vi "solar_addon QTimers.vi"(11 "Variant":variant) -> (0 "error out":errorcluster)   [LabVIEW 2018]
doc: "This SOLAR addon configures the QTimer periodic messaging interface."
uses:
  solar/solar_ctl SOLAR Refnum.ctl
panel:
  in  "Export":bool
  in  "Apply":bool
  in  "Stop All":bool
  out "Destination Queue":string
  in  "Add":bool
  in  "Messages":string
  out "Messages to Enqueue":cluster{"MSG":string, "DATA":variant}[](array[cluster])
  in  "Stop":bool
  in  "Start":bool
  in  "EnQ_Type":enum8{"Normal", "Priority", "IgnoreIfExists"}(ring)
  out "Running":bool
  in  "Delay":i32 format="%d ms"
  out "QTimer":string
  in  "QTimersLB":i32(listbox)
  in  "Refresh":bool
  # "CMD{TYPE:VALUE,...}"
  # "Ex: READ{i32:123,bool:true,str:'test'}"
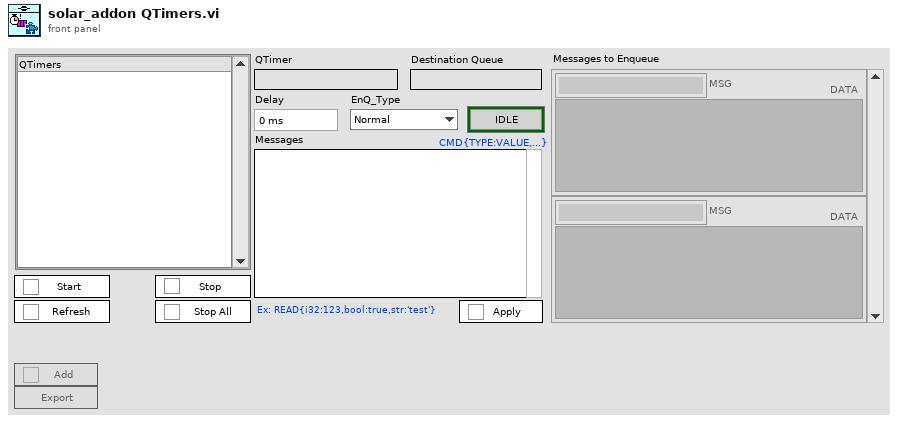
[diagram p1: front panel]
types:
  T1 = typedef "solar_ctl SOLAR Refnum.ctl" = refnum<k1>
  T2 = cluster{"image type":i32, "image depth":i32, "image":u8[], "mask":u8[], "colors":u32[], "Rectangle":cluster{"left":i16, "top":i16, "right":i16, "bottom":i16}}[]
  T3 = typedef "solar_ctl SOLAR Global.ctl" = cluster{"Targets":T4[], "AppDir":path, "solar.ini":path, "ConfigsDir":path, "CosmosDir":path, "LogsDir":path, "ExePath":path, "ExeVersion":string, "PartNum":string, "AppSetup":string, "Title":string, "Main.ini":path, "Temp.ini":path, "vSOLAR":string, "Splash.png":string, "SplashWait":i32, "SOLARUE":refnum<user-event>, "VoyagerRefnum":T5, "QTimerRefnum":T6}
  T4 = typedef "solar_ctl Target Global.ctl" = cluster{"Target":string, "Q":refnum<queue>, "UE":refnum<user-event>, "VI":refnum<vi>, "Menu":refnum<k9>, "Data":refnum<data-value>, "Attributes":variant}
  T5 = typedef "solar_voy_ctl Voyager Refnum.ctl" = refnum<k1>
  T6 = typedef "solar_qtimer_ctl Refnum.ctl" = refnum<k1>
  T7 = typedef "solar_qtimer_ctl QTimer.ctl" = cluster{"Settings":T8, "Queue":refnum<queue>, "QTimerQ":refnum<queue>, "VI Refnum":refnum<vi>}
  T8 = typedef "solar_qtimer_ctl QTimer Settings.ctl" = cluster{"QTimer":string, "Delay":i32, "Start":bool, "EnQ_Type":enum8{"Normal", "Priority", "IgnoreIfExists"}, "Messages":cluster{"MSG":string, "DATA":variant}[]}
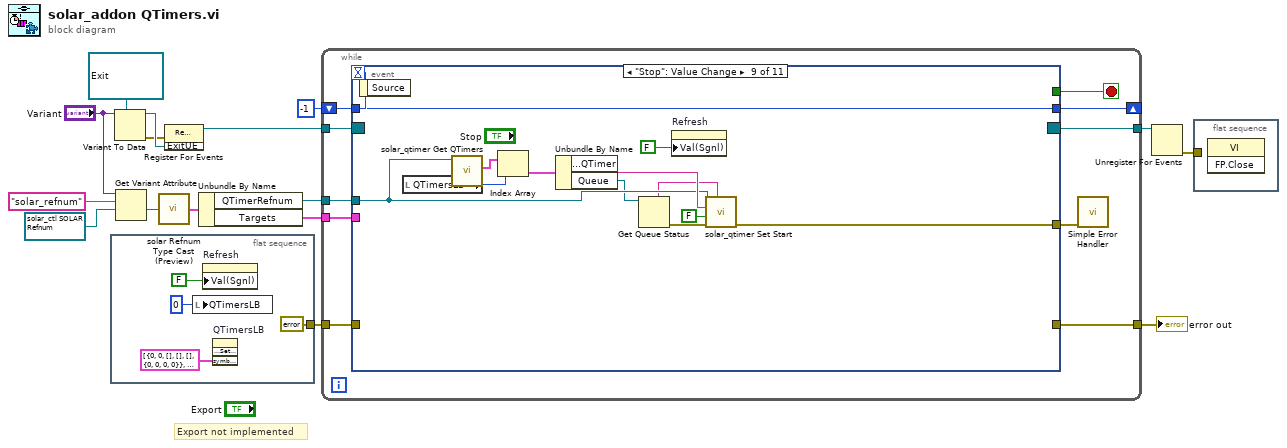
[diagram p0: block diagram]
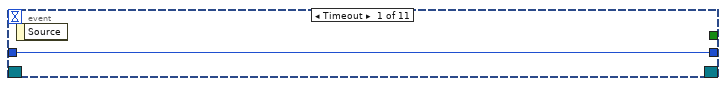
[diagram p2: hidden frame]
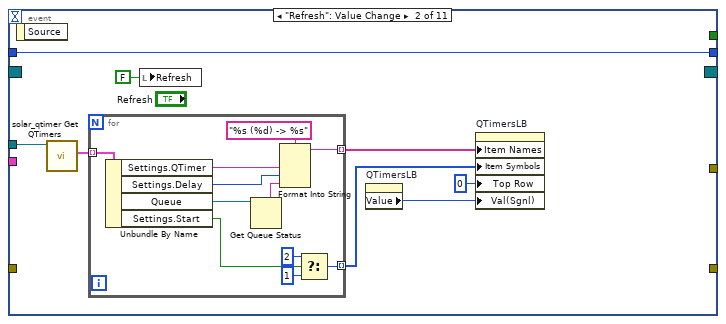
[diagram p3: hidden frame]
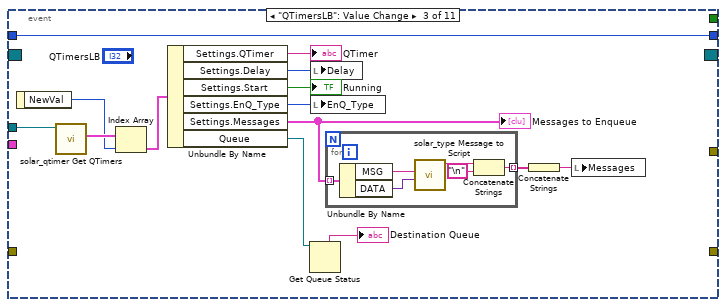
[diagram p4: hidden frame]
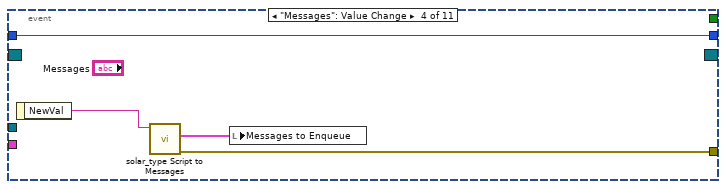
[diagram p5: hidden frame]
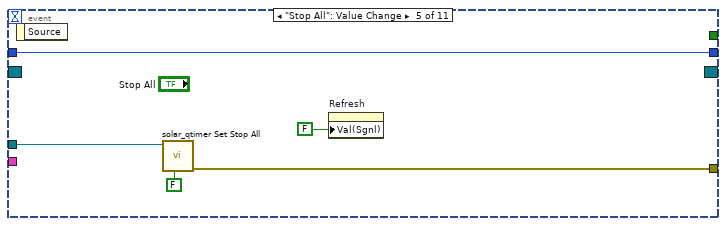
[diagram p6: hidden frame]
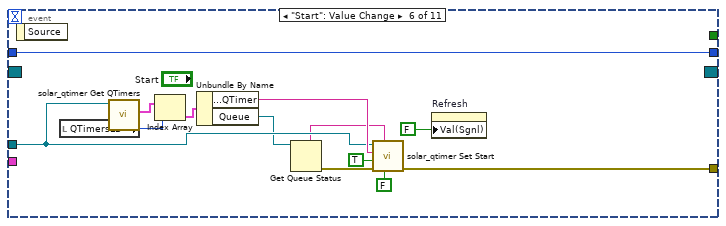
[diagram p7: hidden frame]
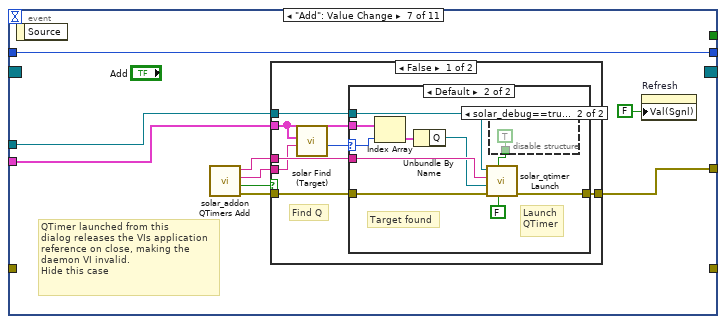
[diagram p8: hidden frame]
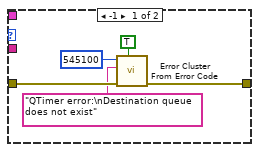
[diagram p9: hidden frame]
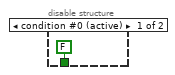
[diagram p10: hidden frame]
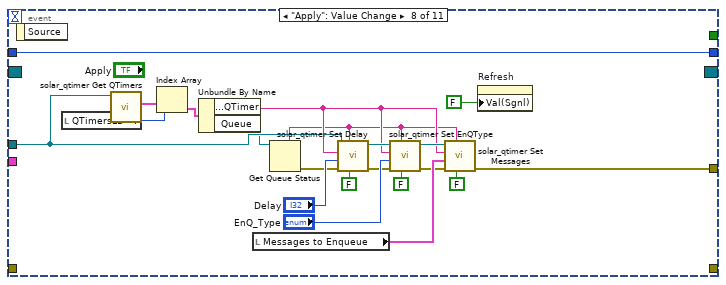
[diagram p12: hidden frame]
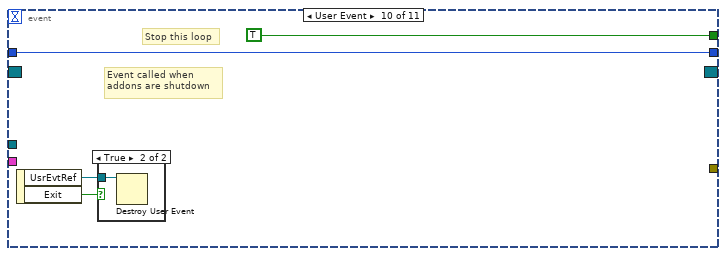
[diagram p13: hidden frame]
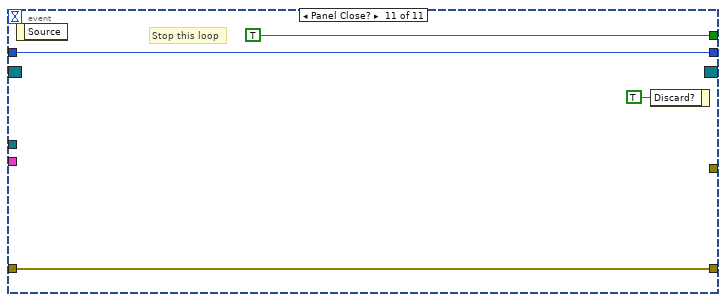
[diagram p15: hidden frame]
diagram:
  w11 = T1 refnum items=["solar"] ("SOLAR Refnum")
  # "Export not implemented"
  n1 = flat-sequence {
    tunnel: [errorcluster {"status"=FALSE, "code"=0, "source"=""} ("error in (no error)")] -> w1
    frame #0 {
      n2 = local write "QTimersLB"(0 ("QTimersLB")) -> ()
      n3 = property on="Refresh" class="Bool (strict)"("Val(Sgnl)"=FALSE ("Update")) -> ()  [unwired: 2 in, 2 out]
      n4 = invoke on="QTimersLB" class="LstBox (strict)" method="Custom Item Symbols.Set Symbol Array"("symbols"=T2 [{"image type"=0, "image depth"=0, "image"=[], "mask"=[], "colors"=[], "Rectangle"={"left"=0, "top"=0, "right"=0, "bottom"=0}}, {"image type"=0, "image depth"=32, "image"=[0, 0, 0, 0, 0, 0, 0, 0, 0, 0, 0, 0, 0, 0, 0, 0, 0, 0, 0, 0, 0, 0, 0, 0, 0, 0, 0, 0, 0, 0, 0, 0, 0, 0, 0, 0, 0, 0, 0, 0, 0, 0, 0, 0, 0, 0, 0, 0, 0, 0, 0, 0, 0, 0, 0, 0, 0, 0, 0, 0, 0, 0, 0, 0, 0, 0, 0, 0, 0, 0, 0, 0, 0, 0, 0, 0, 0, 0, 0, 0, 0, 0, 0, 0, 0, 0, 0, 0, 0, 0, 0, 0, 0, 0, 0, 0, 0, 0, 0, 0, 0, 0, 0, 0, 0, 0, 0, 0, 0, 0, 0, 0, 0, 0, 0, 0, 0, 0, 0, 0, 0, 0, 0, 0, 0, 0, 0, 0, 0, 0, 0, 0, 0, 0, 0, 0, 255, 157, 0, 0, 255, 157, 0, 0, 255, 157, 0, 0, 255, 157, 0, 0, 255, 157, 0, 0, 255, 157, 0, 0, 255, 157, 0, 0, 255, 157, 0, 0, 255, 157, 0, 0, 255, 157, 0, 0, 255, 157, 0, 0, 255, 157, 0, 0, 0, 0, 0, 0, 0, 0, 0, 0, 0, 0, 0, 0, 0, 0, 0, 0, 255, 157, 0, 0, 255, 247, 0, 0, 255, 247, 0, 0, 255, 247, 0, 0, 255, 247, 0, 0, 255, 247, 0, 0, 255, 247, 0, 0, 255, 247, 0, 0, 255, 247, 0, 0, 255, 247, 0, 0, 255, 247, 0, 0, 255, 157, 0, 0, 0, 0, 0, 0, 0, 0, 0, 0, 0, 0, 0, 0, 0, 0, 0, 0, 255, 157, 0, 0, 255, 240, 0, 0, 255, 240, 0, 0, 255, 240, 0, 0, 255, 240, 0, 0, 255, 240, 0, 0, 255, 240, 0, 0, 255, 240, 0, 0, 255, 240, 0, 0, 255, 240, 0, 0, 255, 240, 0, 0, 255, 157, 0, 0, 0, 0, 0, 0, 0, 0, 0, 0, 0, 0, 0, 0, 0, 0, 0, 0, 255, 157, 0, 0, 255, 232, 0, 0, 255, 232, 0, 0, 255, 232, 0, 0, 255, 232, 0, 0, 255, 232, 0, 0, 255, 232, 0, 0, 255, 232, 0, 0, 255, 232, 0, 0, 255, 232, 0, 0, 255, 232, 0, 0, 255, 157, 0, 0, 0, 0, 0, 0, 0, 0, 0, 0, 0, 0, 0, 0, 0, 0, 0, 0, 255, 157, 0, 0, 255, 225, 0, 0, 255, 225, 0, 0, 255, 225, 0, 0, 255, 225, 0, 0, 255, 225, 0, 0, 255, 225, 0, 0, 255, 225, 0, 0, 255, 225, 0, 0, 255, 225, 0, 0, 255, 225, 0, 0, 255, 157, 0, 0, 0, 0, 0, 0, 0, 0, 0, 0, 0, 0, 0, 0, 0, 0, 0, 0, 255, 157, 0, 0, 255, 217, 0, 0, 255, 217, 0, 0, 255, 217, 0, 0, 255, 217, 0, 0, 255, 217, 0, 0, 255, 217, 0, 0, 255, 217, 0, 0, 255, 217, 0, 0, 255, 217, 0, 0, 255, 217, 0, 0, 255, 157, 0, 0, 0, 0, 0, 0, 0, 0, 0, 0, 0, 0, 0, 0, 0, 0, 0, 0, 255, 157, 0, 0, 255, 210, 0, 0, 255, 210, 0, 0, 255, 210, 0, 0, 255, 210, 0, 0, 255, 210, 0, 0, 255, 210, 0, 0, 255, 210, 0, 0, 255, 210, 0, 0, 255, 210, 0, 0, 255, 210, 0, 0, 255, 157, 0, 0, 0, 0, 0, 0, 0, 0, 0, 0, 0, 0, 0, 0, 0, 0, 0, 0, 255, 157, 0, 0, 255, 202, 0, 0, 255, 202, 0, 0, 255, 202, 0, 0, 255, 202, 0, 0, 255, 202, 0, 0, 255, 202, 0, 0, 255, 202, 0, 0, 255, 202, 0, 0, 255, 202, 0, 0, 255, 202, 0, 0, 255, 157, 0, 0, 0, 0, 0, 0, 0, 0, 0, 0, 0, 0, 0, 0, 0, 0, 0, 0, 255, 157, 0, 0, 255, 195, 0, 0, 255, 195, 0, 0, 255, 195, 0, 0, 255, 195, 0, 0, 255, 195, 0, 0, 255, 195, 0, 0, 255, 195, 0, 0, 255, 195, 0, 0, 255, 195, 0, 0, 255, 195, 0, 0, 255, 157, 0, 0, 0, 0, 0, 0, 0, 0, 0, 0, 0, 0, 0, 0, 0, 0, 0, 0, 255, 157, 0, 0, 255, 187, 0, 0, 255, 187, 0, 0, 255, 187, 0, 0, 255, 187, 0, 0, 255, 187, 0, 0, 255, 187, 0, 0, 255, 187, 0, 0, 255, 187, 0, 0, 255, 187, 0, 0, 255, 187, 0, 0, 255, 157, 0, 0, 0, 0, 0, 0, 0, 0, 0, 0, 0, 0, 0, 0, 0, 0, 0, 0, 255, 157, 0, 0, 255, 165, 0, 0, 255, 165, 0, 0, 255, 165, 0, 0, 255, 165, 0, 0, 255, 165, 0, 0, 255, 165, 0, 0, 255, 165, 0, 0, 255, 165, 0, 0, 255, 165, 0, 0, 255, 165, 0, 0, 255, 157, 0, 0, 0, 0, 0, 0, 0, 0, 0, 0, 0, 0, 0, 0, 0, 0, 0, 0, 255, 157, 0, 0, 255, 157, 0, 0, 255, 157, 0, 0, 255, 157, 0, 0, 255, 157, 0, 0, 255, 157, 0, 0, 255, 157, 0, 0, 255, 157, 0, 0, 255, 157, 0, 0, 255, 157, 0, 0, 255, 157, 0, 0, 255, 157, 0, 0, 0, 0, 0, 0, 0, 0, 0, 0, 0, 0, 0, 0, 0, 0, 0, 0, 0, 0, 0, 0, 0, 0, 0, 0, 0, 0, 0, 0, 0, 0, 0, 0, 0, 0, 0, 0, 0, 0, 0, 0, 0, 0, 0, 0, 0, 0, 0, 0, 0, 0, 0, 0, 0, 0, 0, 0, 0, 0, 0, 0, 0, 0, 0, 0, 0, 0, 0, 0, 0, 0, 0, 0, 0, 0, 0, 0, 0, 0, 0, 0, 0, 0, 0, 0, 0, 0, 0, 0, 0, 0, 0, 0, 0, 0, 0, 0, 0, 0, 0, 0, 0, 0, 0, 0, 0, 0, 0, 0, 0, 0, 0, 0, 0, 0, 0, 0, 0, 0, 0, 0, 0, 0, 0, 0, 0, 0, 0, 0, 0, 0, 0, 0, 0, 0, 0, 0], "mask"=[0, 0, 0, 0, 63, 252, 63, 252, 63, 252, 63, 252, 63, 252, 63, 252, 63, 252, 63, 252, 63, 252, 63, 252, 63, 252, 63, 252, 0, 0, 0, 0], "colors"=[], "Rectangle"={"left"=0, "top"=0, "right"=16, "bottom"=16}}, {"image type"=0, "image depth"=32, "image"=[0, 0, 0, 0, 0, 0, 0, 0, 0, 0, 0, 0, 0, 0, 0, 0, 0, 0, 0, 0, 0, 0, 0, 0, 0, 0, 0, 0, 0, 0, 0, 0, 0, 0, 0, 0, 0, 0, 0, 0, 0, 0, 0, 0, 0, 0, 0, 0, 0, 0, 0, 0, 0, 0, 0, 0, 0, 0, 0, 0, 0, 0, 0, 0, 0, 0, 0, 0, 0, 0, 0, 0, 0, 0, 0, 0, 0, 0, 0, 0, 255, 0, 102, 0, 255, 0, 102, 0, 255, 0, 102, 0, 0, 0, 0, 0, 0, 0, 0, 0, 0, 0, 0, 0, 0, 0, 0, 0, 0, 0, 0, 0, 0, 0, 0, 0, 0, 0, 0, 0, 0, 0, 0, 0, 0, 0, 0, 0, 0, 0, 0, 0, 0, 0, 0, 0, 0, 0, 0, 0, 0, 0, 0, 0, 255, 0, 102, 0, 255, 133, 241, 88, 255, 133, 241, 88, 255, 0, 102, 0, 0, 0, 0, 0, 0, 0, 0, 0, 0, 0, 0, 0, 0, 0, 0, 0, 0, 0, 0, 0, 0, 0, 0, 0, 0, 0, 0, 0, 0, 0, 0, 0, 0, 0, 0, 0, 0, 0, 0, 0, 0, 0, 0, 0, 0, 0, 0, 0, 255, 0, 102, 0, 255, 122, 235, 82, 255, 122, 235, 82, 255, 122, 235, 82, 255, 0, 102, 0, 0, 0, 0, 0, 0, 0, 0, 0, 0, 0, 0, 0, 0, 0, 0, 0, 0, 0, 0, 0, 0, 0, 0, 0, 0, 0, 0, 0, 0, 0, 0, 0, 0, 0, 0, 0, 0, 0, 0, 0, 0, 0, 0, 0, 255, 0, 102, 0, 255, 112, 228, 75, 255, 112, 228, 75, 255, 112, 228, 75, 255, 112, 228, 75, 255, 0, 102, 0, 0, 0, 0, 0, 0, 0, 0, 0, 0, 0, 0, 0, 0, 0, 0, 0, 0, 0, 0, 0, 0, 0, 0, 0, 0, 0, 0, 0, 0, 0, 0, 0, 0, 0, 0, 0, 0, 0, 0, 0, 255, 0, 102, 0, 255, 102, 221, 68, 255, 102, 221, 68, 255, 102, 221, 68, 255, 102, 221, 68, 255, 102, 221, 68, 255, 0, 102, 0, 0, 0, 0, 0, 0, 0, 0, 0, 0, 0, 0, 0, 0, 0, 0, 0, 0, 0, 0, 0, 0, 0, 0, 0, 0, 0, 0, 0, 0, 0, 0, 0, 0, 0, 0, 0, 255, 0, 101, 0, 255, 92, 214, 61, 255, 92, 214, 61, 255, 92, 214, 61, 255, 92, 214, 61, 255, 92, 214, 61, 255, 92, 214, 61, 255, 0, 102, 0, 0, 0, 0, 0, 0, 0, 0, 0, 0, 0, 0, 0, 0, 0, 0, 0, 0, 0, 0, 0, 0, 0, 0, 0, 0, 0, 0, 0, 0, 0, 0, 0, 255, 0, 101, 0, 255, 82, 207, 54, 255, 82, 207, 54, 255, 82, 207, 54, 255, 82, 207, 54, 255, 82, 207, 54, 255, 82, 207, 54, 255, 82, 207, 54, 255, 0, 102, 0, 0, 0, 0, 0, 0, 0, 0, 0, 0, 0, 0, 0, 0, 0, 0, 0, 0, 0, 0, 0, 0, 0, 0, 0, 0, 0, 0, 0, 255, 0, 102, 0, 255, 71, 201, 48, 255, 71, 201, 48, 255, 71, 201, 48, 255, 71, 201, 48, 255, 71, 201, 48, 255, 71, 201, 48, 255, 71, 201, 48, 255, 0, 102, 0, 0, 0, 0, 0, 0, 0, 0, 0, 0, 0, 0, 0, 0, 0, 0, 0, 0, 0, 0, 0, 0, 0, 0, 0, 0, 0, 0, 0, 255, 0, 102, 0, 255, 61, 194, 41, 255, 61, 194, 41, 255, 61, 194, 41, 255, 61, 194, 41, 255, 61, 194, 41, 255, 61, 194, 41, 255, 0, 102, 0, 0, 0, 0, 0, 0, 0, 0, 0, 0, 0, 0, 0, 0, 0, 0, 0, 0, 0, 0, 0, 0, 0, 0, 0, 0, 0, 0, 0, 0, 0, 0, 0, 255, 0, 101, 0, 255, 51, 187, 34, 255, 51, 187, 34, 255, 51, 187, 34, 255, 51, 187, 34, 255, 51, 187, 34, 255, 0, 102, 0, 0, 0, 0, 0, 0, 0, 0, 0, 0, 0, 0, 0, 0, 0, 0, 0, 0, 0, 0, 0, 0, 0, 0, 0, 0, 0, 0, 0, 0, 0, 0, 0, 0, 0, 0, 0, 255, 0, 102, 0, 255, 41, 180, 27, 255, 41, 180, 27, 255, 41, 180, 27, 255, 41, 180, 27, 255, 0, 102, 0, 0, 0, 0, 0, 0, 0, 0, 0, 0, 0, 0, 0, 0, 0, 0, 0, 0, 0, 0, 0, 0, 0, 0, 0, 0, 0, 0, 0, 0, 0, 0, 0, 0, 0, 0, 0, 0, 0, 0, 0, 255, 0, 102, 0, 255, 31, 173, 20, 255, 31, 173, 20, 255, 31, 173, 20, 255, 0, 102, 0, 0, 0, 0, 0, 0, 0, 0, 0, 0, 0, 0, 0, 0, 0, 0, 0, 0, 0, 0, 0, 0, 0, 0, 0, 0, 0, 0, 0, 0, 0, 0, 0, 0, 0, 0, 0, 0, 0, 0, 0, 0, 0, 0, 0, 255, 0, 102, 0, 255, 20, 167, 14, 255, 20, 167, 14, 255, 0, 102, 0, 0, 0, 0, 0, 0, 0, 0, 0, 0, 0, 0, 0, 0, 0, 0, 0, 0, 0, 0, 0, 0, 0, 0, 0, 0, 0, 0, 0, 0, 0, 0, 0, 0, 0, 0, 0, 0, 0, 0, 0, 0, 0, 0, 0, 0, 0, 0, 0, 255, 0, 102, 0, 255, 0, 102, 0, 255, 0, 102, 0, 0, 0, 0, 0, 0, 0, 0, 0, 0, 0, 0, 0, 0, 0, 0, 0, 0, 0, 0, 0, 0, 0, 0, 0, 0, 0, 0, 0, 0, 0, 0, 0, 0, 0, 0, 0, 0, 0, 0, 0, 0, 0, 0, 0, 0, 0, 0, 0, 0, 0, 0, 0, 0, 0, 0, 0, 0, 0, 0, 0, 0, 0, 0, 0, 0, 0, 0, 0, 0, 0, 0, 0, 0, 0, 0, 0, 0, 0, 0, 0, 0, 0, 0, 0, 0, 0, 0, 0, 0, 0, 0, 0, 0, 0, 0, 0, 0, 0, 0, 0], "mask"=[0, 0, 14, 0, 15, 0, 15, 128, 15, 192, 15, 224, 15, 240, 15, 248, 15, 248, 15, 240, 15, 224, 15, 192, 15, 128, 15, 0, 14, 0, 0, 0], "colors"=[], "Rectangle"={"left"=0, "top"=0, "right"=16, "bottom"=16}}] ("Symbols")) -> ()  [unwired: 3 in, 4 out]
    }
  }
  n5 = Variant To Data(type=refnum<user-event> refnum ("ExitUE"), Variant="Variant") -> (data=w13:refnum<user-event>, error out=w12:errorcluster)  [unwired: 1 in]
  n6 = Get Variant Attribute(Variant="Variant", name="solar_refnum", default value (empty Variant)=w11) -> (value=w7:T1)  [unwired: 1 in, 3 out]
  n7 = call "solar Refnum Type Cast (Preview).vi"("Refnum"=w7) -> ("SOLAR"=w8:T3)  [unwired: 8 in]
  n8 = register-events(error in=w12, w13) -> (reference out=w15:refnum<event-registration>)  [unwired: 1 in, 1 out]
  n9 = Unbundle By Name(w8) -> ("QTimerRefnum"=w6:T6, "Targets"=w5:T4[])
  n10 = while {
    tunnel: w15 -> [w30]
    shift-right: [w28] -> _
    shift-left: -1 -> [w27]
    tunnel: w6 -> [w26]
    tunnel: w5 -> [w24]
    tunnel: [w23] -> w4
    tunnel: [w22] -> w2
    tunnel: w1 -> [w21]
    stop <- w29 stop-if-true
    n11 = event shown="[8] \"Stop\": Value Change" {
      selector: w30 -> [_ _ _ _ _ _ _ _ _ _ _]
      dyn-events: [_ _ _ _ _ _ _ _ _ _ _] -> w23
      timeout: w27 -> [_ _ _ _ _ _ _ _ _ _ _]
      tunnel: [_ _ _ _ _ _ _ _ _ TRUE TRUE] -> w29
      tunnel: [w31 w39 w64 w74 w79 w92 w101 w147 w159 w162 w167] -> w28
      tunnel: w27 -> [w31 w39 w64 w74 w79 w92 w101 w147 w159 w162 w167]
      tunnel: w26 -> [_ w33 w63 _ w78 w82 w100 w130 w151 _ _]
      tunnel: [_ _ _ w72 w76 w88 w94 w136 w154 _ _] -> w25
      tunnel: w24 -> [_ _ _ _ _ _ w93 _ _ _ _]
      tunnel: [_ _ _ _ _ _ _ _ _ _ w165] -> w22
      tunnel: w21 -> [_ _ _ _ _ _ _ _ _ _ w165]
      event Timeout {
        n12 = event-data() -> ()  [unwired: 1 in, 1 out]
      }
      event "Refresh": Value Change {
        n13 = event-data() -> ()  [unwired: 1 in, 1 out]
        n14 = call "solar_qtimer Get QTimers.vi"("QTimer Refnum"=w33) -> ("QTimers"=w37:T7[])  [unwired: 8 in, 2 out]
        n15 = for {
          tunnel: w37 -> [w50] mode=indexing
          tunnel: [w43] -> w36 mode=indexing
          tunnel: [w42] -> w35 mode=indexing
          n16 = Unbundle By Name(w50) -> ("Settings.QTimer"=w49:string, "Settings.Delay"=w44:i32, "Queue"=w41:refnum<queue>, "Settings.Start"=w47:bool)
          n17 = Get Queue Status(queue=w41) -> (queue name=w40:string)  [unwired: 2 in, 7 out]
          n18 = Format Into String(format string="%s (%d) -> %s", w49, w44, w40) -> (resulting string=w43:string)  [unwired: 2 in, 1 out]
          n19 = Select(t=2, s=w47, f=1) -> (s? t:f=w42:i32)
        }
        n20 = local write "Refresh"(FALSE ("Update")) -> ()
        n21 = property on="QTimersLB" class="LstBox (strict)"() -> ("Value"=w32:i32)  [unwired: 2 in, 2 out]
        n22 = property on="QTimersLB" class="LstBox (strict)"("Item Names"=w36, "Item Symbols"=w35, "Top Row"=0, "Val(Sgnl)"=w32) -> ()  [unwired: 2 in, 2 out]
      }
      event "QTimersLB": Value Change {
        n23 = event-data() -> ("NewVal"=w61:i32)  [unwired: 1 in]
        n24 = call "solar_qtimer Get QTimers.vi"("QTimer Refnum"=w63) -> ("QTimers"=w62:T7[])  [unwired: 8 in, 2 out]
        n25 = Index Array(array=w62, index=w61) -> (element=w60:T7)
        n26 = Unbundle By Name(w60) -> ("Settings.QTimer"=→"QTimer":string, "Settings.Delay"=w58:i32, "Settings.Start"=→"Running":bool, "Settings.EnQ_Type"=w57:enum8{"Normal", "Priority", "IgnoreIfExists"}, "Settings.Messages"=w53:cluster{"MSG":string, "DATA":variant}[], "Queue"=w56:refnum<queue>)
        "Messages to Enqueue" <- w53
        n27 = Get Queue Status(queue=w56) -> (queue name=→"Destination Queue":string)  [unwired: 2 in, 7 out]
        n28 = local write "Delay"(w58) -> ()
        n29 = local write "EnQ_Type"(w57) -> ()
        n30 = for {
          tunnel: w53 -> [w70] mode=indexing
          tunnel: [w66] -> w52 mode=indexing
          n31 = Unbundle By Name(w70) -> ("MSG"=w69:string, "DATA"=w68:variant)
          n32 = call "solar_type Message to Script.vi"("Data"=w68, "Packet"=w69) -> ("String"=w67:string)  [unwired: 8 in, 1 out]
          n33 = Concatenate Strings(w67, "\n" ("Line Feed Constant")) -> (w66:string)
        }
        n34 = Concatenate Strings(w52) -> (w51:string)
        n35 = local write "Messages"(w51) -> ()
      }
      event "Messages": Value Change {
        n36 = event-data() -> ("NewVal"=w73:string)  [unwired: 1 in]
        n37 = call "solar_type Script to Messages.vi"("Script String"=w73) -> ("error out"=w72:errorcluster, "Messages"=w71:cluster{"MSG":string, "DATA":variant}[])  [unwired: 7 in, 2 out]
        n38 = local write "Messages to Enqueue"(w71) -> ()
      }
      event "Stop All": Value Change {
        n39 = event-data() -> ()  [unwired: 1 in, 1 out]
        n40 = call "solar_qtimer Set Stop All.vi"("Suppress Errors? (T)"=FALSE, "QTimer Refnum in"=w78) -> ("error out"=w76:errorcluster)  [unwired: 6 in, 3 out]
        n41 = property on="Refresh" class="Bool (strict)"("Val(Sgnl)"=FALSE ("Update")) -> ()  [unwired: 2 in, 2 out]
      }
      event "Start": Value Change {
        n42 = event-data() -> ()  [unwired: 1 in, 1 out]
        n43 = local read "QTimersLB"() -> (w89:i32)
        n44 = call "solar_qtimer Get QTimers.vi"("QTimer Refnum"=w82) -> ("QTimers"=w86:T7[])  [unwired: 8 in, 2 out]
        n45 = Index Array(array=w86, index=w89) -> (element=w85:T7)
        n46 = Unbundle By Name(w85) -> ("Settings.QTimer"=w84:string, "Queue"=w81:refnum<queue>)
        n47 = Get Queue Status(queue=w81) -> (queue name=w80:string, error out=w83:errorcluster)  [unwired: 2 in, 6 out]
        n48 = call "solar_qtimer Set Start.vi"("Suppress Errors? (T)"=FALSE, "Target Name"=w80, "error in (no error)"=w83, "Start (F = Stop)"=TRUE, "QTimer Name"=w84, "QTimer Refnum in"=w82) -> ("error out"=w88:errorcluster)  [unwired: 4 in, 1 out]
        n49 = property on="Refresh" class="Bool (strict)"("Val(Sgnl)"=FALSE ("Update")) -> ()  [unwired: 2 in, 2 out]
      }
      event "Add": Value Change {
        # "QTimer launched from this\ndialog releases the VIs application\nreference on close, making the \ndaemon VI invalid.\nHide this case"
        n50 = event-data() -> ()  [unwired: 1 in, 1 out]
        n51 = call "solar_addon QTimers Add.vi"() -> ("error out"=w98:errorcluster, "Cancelled"=w95:bool, "Target out"=w97:string, "QTimer out"=w99:string)  [unwired: 8 in]
        n52 = case shown="False" w95 {
          tunnel: w100 -> [w108 _]
          tunnel: w99 -> [w107 _]
          tunnel: w98 -> [w102 w126]
          tunnel: w97 -> [w105 _]
          tunnel: [w106 w126] -> w94
          tunnel: w93 -> [w104 _]
          frame False {
            # "Find Q"
            n53 = call "solar Find (Target).vi"("Target"=w105, "Targets"=w104) -> ("Target Index"=w103:i32)  [unwired: 8 in, 1 out]
            n54 = case shown="Default" w103 {
              selector: w103 -> [_ w118]
              tunnel: w108 -> [_ w123]
              tunnel: w107 -> [_ w122]
              tunnel: [w112 w121] -> w106
              tunnel: w104 -> [_ w119]
              tunnel: w102 -> [w113 w116]
              frame -1 {
                n55 = call <vilib>:"Error Cluster From Error Code.vi"("show call chain? (False)"=TRUE, "error in (no error)"=w113, "error message (\"\")"="QTimer error:\nDestination queue does not exist" ("error message (\"\")"), "error code (0)"=545100) -> ("error out"=w112:errorcluster)  [unwired: 5 in]
              }
              frame Default {
                # "Launch\nQTimer"
                # "Target found"
                n56 = Index Array(array=w119, index=w118) -> (element=w117:T4)
                n57 = Unbundle By Name(w117) -> ("Q"=w115:refnum<queue>)
                n58 = disable-structure shown="solar_debug==true" {
                  disable-tunnel: [FALSE TRUE ("Open FP? (F)")] -> w114
                  frame condition #0 (active) {
                  }
                  frame condition #1 {
                  }
                }
                n59 = call "solar_qtimer Launch.vi"("Suppress Errors? (T)"=FALSE, "Open FP? (F)"=w114, "error in (no error)"=w116, "Target Queue"=w115, "QTimer Name"=w122, "QTimer Refnum in"=w123) -> ("error out"=w121:errorcluster)  [unwired: 4 in, 1 out]
              }
            }
          }
          frame True {
            # "Cancelled"
          }
        }
        n60 = property on="Refresh" class="Bool (strict)"("Val(Sgnl)"=FALSE ("Update")) -> ()  [unwired: 2 in, 2 out]
      }
      event "Apply": Value Change {
        n61 = event-data() -> ()  [unwired: 1 in, 1 out]
        n62 = local read "QTimersLB"() -> (w146:i32)
        n63 = call "solar_qtimer Get QTimers.vi"("QTimer Refnum"=w130) -> ("QTimers"=w132:T7[])  [unwired: 8 in, 2 out]
        n64 = Index Array(array=w132, index=w146) -> (element=w140:T7)
        n65 = Unbundle By Name(w140) -> ("Settings.QTimer"=w131:string, "Queue"=w128:refnum<queue>)
        n66 = local read "Messages to Enqueue"() -> (w139:cluster{"MSG":string, "DATA":variant}[])
        n67 = Get Queue Status(queue=w128) -> (queue name=w127:string, error out=w129:errorcluster)  [unwired: 2 in, 6 out]
        n68 = call "solar_qtimer Set Delay.vi"("Suppress Errors? (T)"=FALSE, "Target Name"=w127, "error in (no error)"=w129, "Delay (-1)"="Delay", "QTimer Name"=w131, "QTimer Refnum in"=w130) -> ("error out"=w138:errorcluster, "QTimer Refnum out"=w143:T6)  [unwired: 4 in]
        n69 = call "solar_qtimer Set EnQType.vi"("Suppress Errors? (T)"=FALSE, "Target Name"=w127, "error in (no error)"=w138, "EnQ_Type (IgnoreIfExists)"="EnQ_Type", "QTimer Name"=w131, "QTimer Refnum in"=w143) -> ("error out"=w137:errorcluster, "QTimer Refnum out"=w141:T6)  [unwired: 4 in]
        n70 = call "solar_qtimer Set Messages.vi"("Suppress Errors? (T)"=FALSE, "Target Name"=w127, "error in (no error)"=w137, "Messages"=w139, "QTimer Name"=w131, "QTimer Refnum in"=w141) -> ("error out"=w136:errorcluster)  [unwired: 4 in, 1 out]
        n71 = property on="Refresh" class="Bool (strict)"("Val(Sgnl)"=FALSE ("Update")) -> ()  [unwired: 2 in, 2 out]
      }
      event "Stop": Value Change {
        n72 = event-data() -> ()  [unwired: 1 in, 1 out]
        n73 = local read "QTimersLB"() -> (w156:i32)
        n74 = call "solar_qtimer Get QTimers.vi"("QTimer Refnum"=w151) -> ("QTimers"=w153:T7[])  [unwired: 8 in, 2 out]
        n75 = Index Array(array=w153, index=w156) -> (element=w155:T7)
        n76 = Unbundle By Name(w155) -> ("Settings.QTimer"=w152:string, "Queue"=w149:refnum<queue>)
        n77 = Get Queue Status(queue=w149) -> (queue name=w148:string, error out=w150:errorcluster)  [unwired: 2 in, 6 out]
        n78 = property on="Refresh" class="Bool (strict)"("Val(Sgnl)"=FALSE ("Update")) -> ()  [unwired: 2 in, 2 out]
        n79 = call "solar_qtimer Set Start.vi"("Target Name"=w148, "error in (no error)"=w150, "Start (F = Stop)"=FALSE, "QTimer Name"=w152, "QTimer Refnum in"=w151) -> ("error out"=w154:errorcluster)  [unwired: 5 in, 1 out]
      }
      event User Event {
        # "Stop this loop"
        # "Event called when\naddons are shutdown"
        n80 = event-data() -> ("UsrEvtRef"=w161:refnum<user-event>, "Exit"=w160:bool)  [unwired: 1 in]
        n81 = case shown="True" w160 {
          tunnel: w161 -> [_ w164]
          frame False {
          }
          frame True {
            n82 = Destroy User Event(user event=w164) -> ()  [unwired: 1 in, 1 out]
          }
        }
      }
      event Panel Close? {
        # "Stop this loop"
        n83 = event-data() -> ()  [unwired: 1 in, 1 out]
        n84 = event-data("Discard?"=TRUE) -> ()  [unwired: 1 in, 1 out]
      }
    }
    n85 = call <vilib>:"Simple Error Handler.vi"("error in (no error)"=w25) -> ()  [unwired: 4 in, 5 out]
  }
  "error out" <- w2
  n86 = Unregister For Events(event registration refnum=w4) -> (error out=w3:errorcluster)  [unwired: 1 in]
  n87 = flat-sequence {
    tunnel: w3 -> [_]
    frame #0 {
      n88 = invoke class="VI" method="FP.Close"() -> ()  [unwired: 3 in, 3 out]
    }
  }
